vi "Array elements (not empty).vi"(11 "1D array":string[](array[string])) -> (7 "# elements":i32)   [LabVIEW 2012]
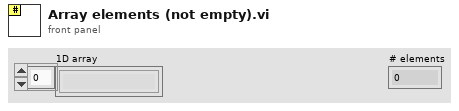
[diagram p1: front panel]
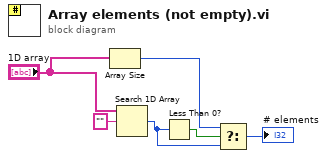
[diagram p0: block diagram]
diagram:
  n1 = Array Size(array="1D array") -> (size(s)=w3:i32)
  n2 = Search 1D Array(1D array="1D array", element="") -> (index of element=w2:i32)  [unwired: 1 in]
  n3 = Less Than 0?(x=w2) -> (x < 0?=w4:bool)
  n4 = Select(t=w3, s=w4, f=w2) -> (s? t:f=→"# elements":i32)
